vi "Read Relay Names.vi"(8 "error in":errorcluster, 11 "2575 in":refnum<class "2575.lvclass">) -> (0 "error out":errorcluster, 3 "2575 out":refnum<class "2575.lvclass">)   [LabVIEW 2019, in "2575.lvlib" / "2575.lvclass"]
uses:
  Library/2575.lvclass
  Library/2575.lvclass/2575.ctl
  Accessors/Read Local Resource.vi
  Accessors/Write Local Resource.vi
  Accessors/Write Device Relay Name.vi
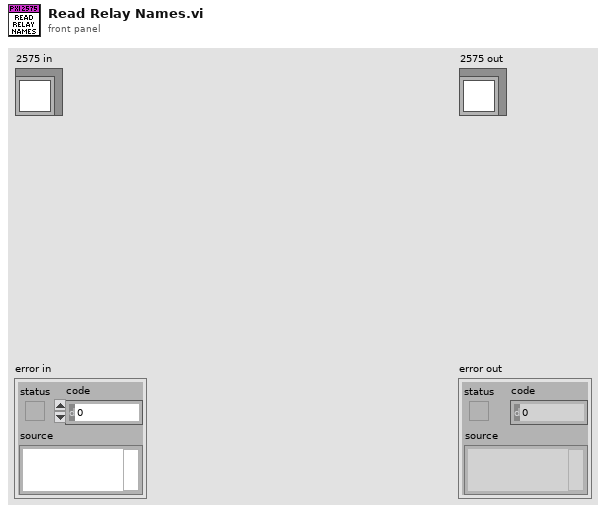
[diagram p1: front panel]
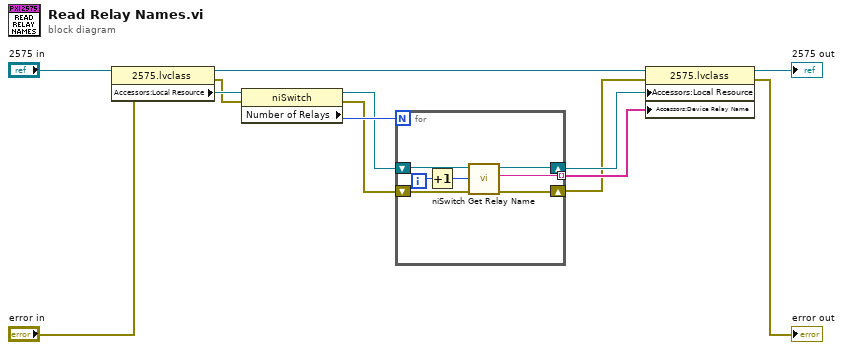
[diagram p0: block diagram]
diagram:
  n1 = property class="2575.lvclass"(reference="2575 in", error in="error in") -> (reference out=w9:refnum<class "2575.lvclass">, error out=w3:errorcluster, "Accessors:Local Resource"=w12:refnum<k15>)
  n2 = property class="niSwitch"(reference=w12, error in=w3) -> (reference out=w10:refnum<k15>, error out=w2:errorcluster, "Number of Relays"=w11:i32)
  n3 = for {
    N: w11 -> [_]
    shift-right: [w19] -> w7
    shift-left: w10 -> [w20]
    tunnel: [w16] -> w6 mode=indexing
    shift-right: [w15] -> w1
    shift-left: w2 -> [w14]
    i -> [w17]
    n4 = Increment(x=w17) -> (x+1=w18:i32)
    n5 = call <instrlib>:"niSwitch Get Relay Name.vi"("error in (no error)"=w14, "index (1)"=w18, "instrument handle"=w20) -> ("error out"=w15:errorcluster, "relay name"=w16:string, "instrument handle out"=w19:refnum<k15>)  [unwired: 6 in]
  }
  n6 = property class="2575.lvclass"(reference=w9, error in=w1, "Accessors:Local Resource"=w7, "Accessors:Device Relay Name"=w6) -> (reference out=→"2575 out":refnum<class "2575.lvclass">, error out=→"error out":errorcluster)
